vi "Close.vi"(8 "error in":errorcluster, 11 "state in":T1) -> (0 "error out":errorcluster)   [LabVIEW 2010, in "NI_SE_Config Front Panel Layout.lvlib"]
uses:
  NI_SE_Config Front Panel Layout.lvlib
  State.ctl
  VI Info.ctl
  VI Panel Layout/VI Panel Layout.lvclass
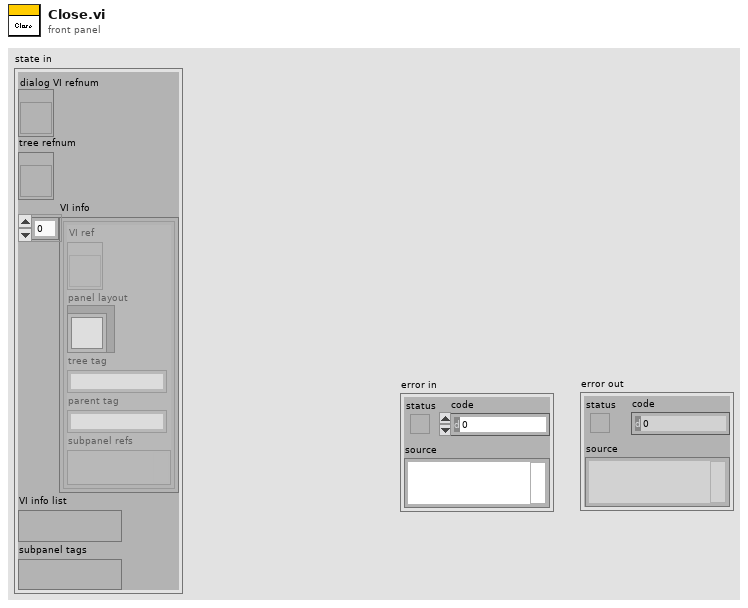
[diagram p1: front panel]
types:
  T1 = typedef "NI_SE_Config Front Panel Layout.lvlib/State.ctl" = cluster{"dialog VI refnum":refnum<vi>, "tree refnum":refnum<vi>, "VI info":T2[], "VI info list":variant, "subpanel tags":variant}
  T2 = typedef "NI_SE_Config Front Panel Layout.lvlib/VI Info.ctl" = cluster{"VI ref":refnum<vi>, "panel layout":refnum<class "VI Panel Layout.lvclass">, "tree tag":string, "parent tag":string, "subpanel refs":variant}
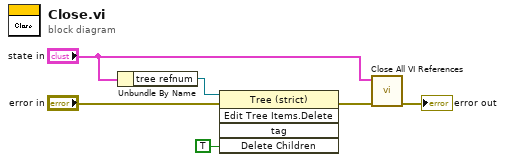
[diagram p0: block diagram]
diagram:
  n1 = Unbundle By Name("state in") -> ("tree refnum"=w3:refnum<vi>)
  n2 = invoke class="Tree (strict)" method="Edit Tree Items.Delete"(reference=w3, error in="error in", "Delete Children"=TRUE ("Delete Children?")) -> (error out=w1:errorcluster)  [unwired: 2 in, 4 out]
  n3 = call "Close All VI References.vi"("error in"=w1, "state in"="state in") -> ("error out"=→"error out":errorcluster)  [unwired: 9 in]
